vi "SaveGraphData.vi"(8 "error in (no error)":errorcluster, 11 "Generador de Funciones in":refnum<class "Generador de Funciones.lvclass">) -> (0 "error out":errorcluster, 3 "Generador de Funciones out":refnum<class "Generador de Funciones.lvclass">)   [LabVIEW 2020, in "Generador de Funciones.lvlib" / "Generador de Funciones.lvclass"]
uses:
  Generador de Funciones.lvclass
  Generador de Funciones.lvclass/Generador de Funciones.ctl
  Loggin/Loggin Messages/saveDAta Msg/saveDAta Msg.lvclass/saveDAta Msg.ctl
  <vilib>/ActorFramework/Message Enqueuer/Message Enqueuer.lvclass/Message Enqueuer.ctl
  <vilib>/ActorFramework/Message Enqueuer/Enqueue.vi
  Loggin/Loggin Messages/saveDAta Msg/saveDAta Msg.lvclass
  C:/Program Files (x86)/National Instruments/LabVIEW 2020/vi.lib/ActorFramework/Message/Message.lvclass
  <vilib>/ActorFramework/Message Priority Queue/Priority Enqueue.vi
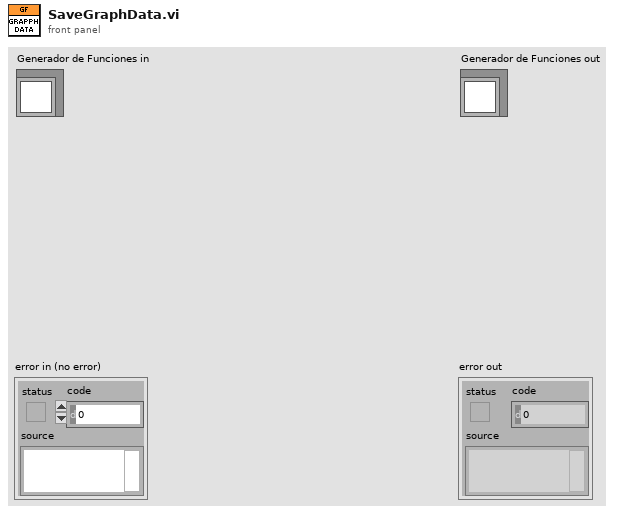
[diagram p1: front panel]
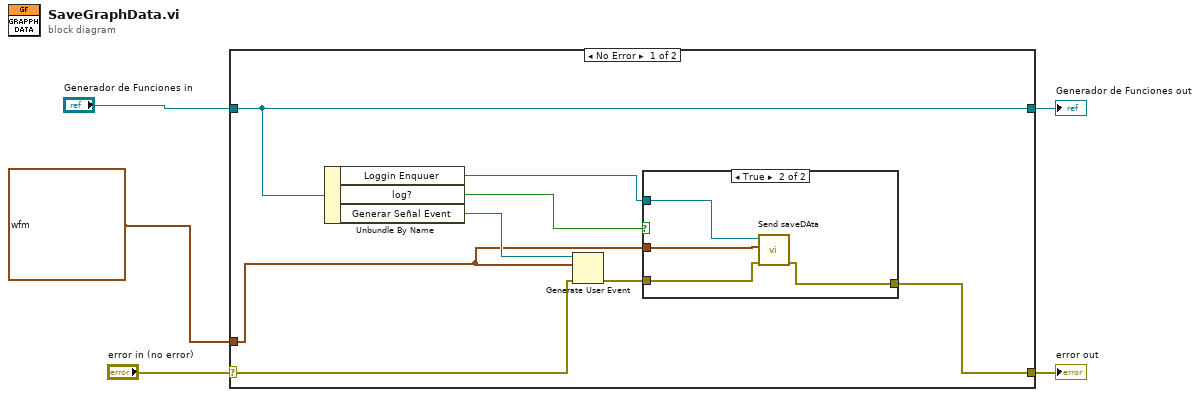
[diagram p0: block diagram]
diagram:
  n1 = case shown="No Error" "error in (no error)" {
    selector: "error in (no error)" -> [w12 w20]
    tunnel: [w8 w20] -> w4
    tunnel: [w13 w19] -> w2
    tunnel: "Generador de Funciones in" -> [w13 w19]
    tunnel: waveform(dbl) {"t0"=timestamp(0 s since 1904-01-01), "dt"=1.0, "Y"=[]} ("Waveform") -> [w7 _]
    frame No Error {
      n2 = Unbundle By Name(w13) -> ("Loggin Enquuer"=w6:refnum<class "Message Enqueuer.lvclass">, "log?"=w10:bool, "Generar Señal Event"=w11:refnum<user-event>)
      n3 = Generate User Event(user event=w11, event data cluster=w7, error in=w12) -> (error out=w9:errorcluster)  [unwired: 1 in, 1 out]
      n4 = case shown="True" w10 {
        tunnel: [w14 w18] -> w8
        tunnel: w9 -> [w14 w17]
        tunnel: w7 -> [_ w16]
        tunnel: w6 -> [_ w15]
        frame False {
        }
        frame True {
          n5 = call "Send saveDAta.vi"("error in (no error)"=w17, "Numeric"=w16, "Message Enqueuer"=w15) -> ("error out"=w18:errorcluster)  [unwired: 7 in, 1 out]
        }
      }
    }
    frame Error {
    }
  }
  "error out" <- w4
  "Generador de Funciones out" <- w2
